vi "Analysis_Main.vi"() -> ()   [LabVIEW 2018]
uses:
  <vilib>/Utility/file.llb/Read Delimited Spreadsheet (string).vi
panel:
  in  "Path":path
  out "Duty":dbl format="%#_g %"
  out "Frequency":dbl format="%#_g Hz"
  out "DeltaT":dbl format="%#_g ms"
  in  "stop":bool
  out "Cursor 2":dbl
  out "Cursor 1":dbl
  out "Data":waveform(dbl)[](graph)
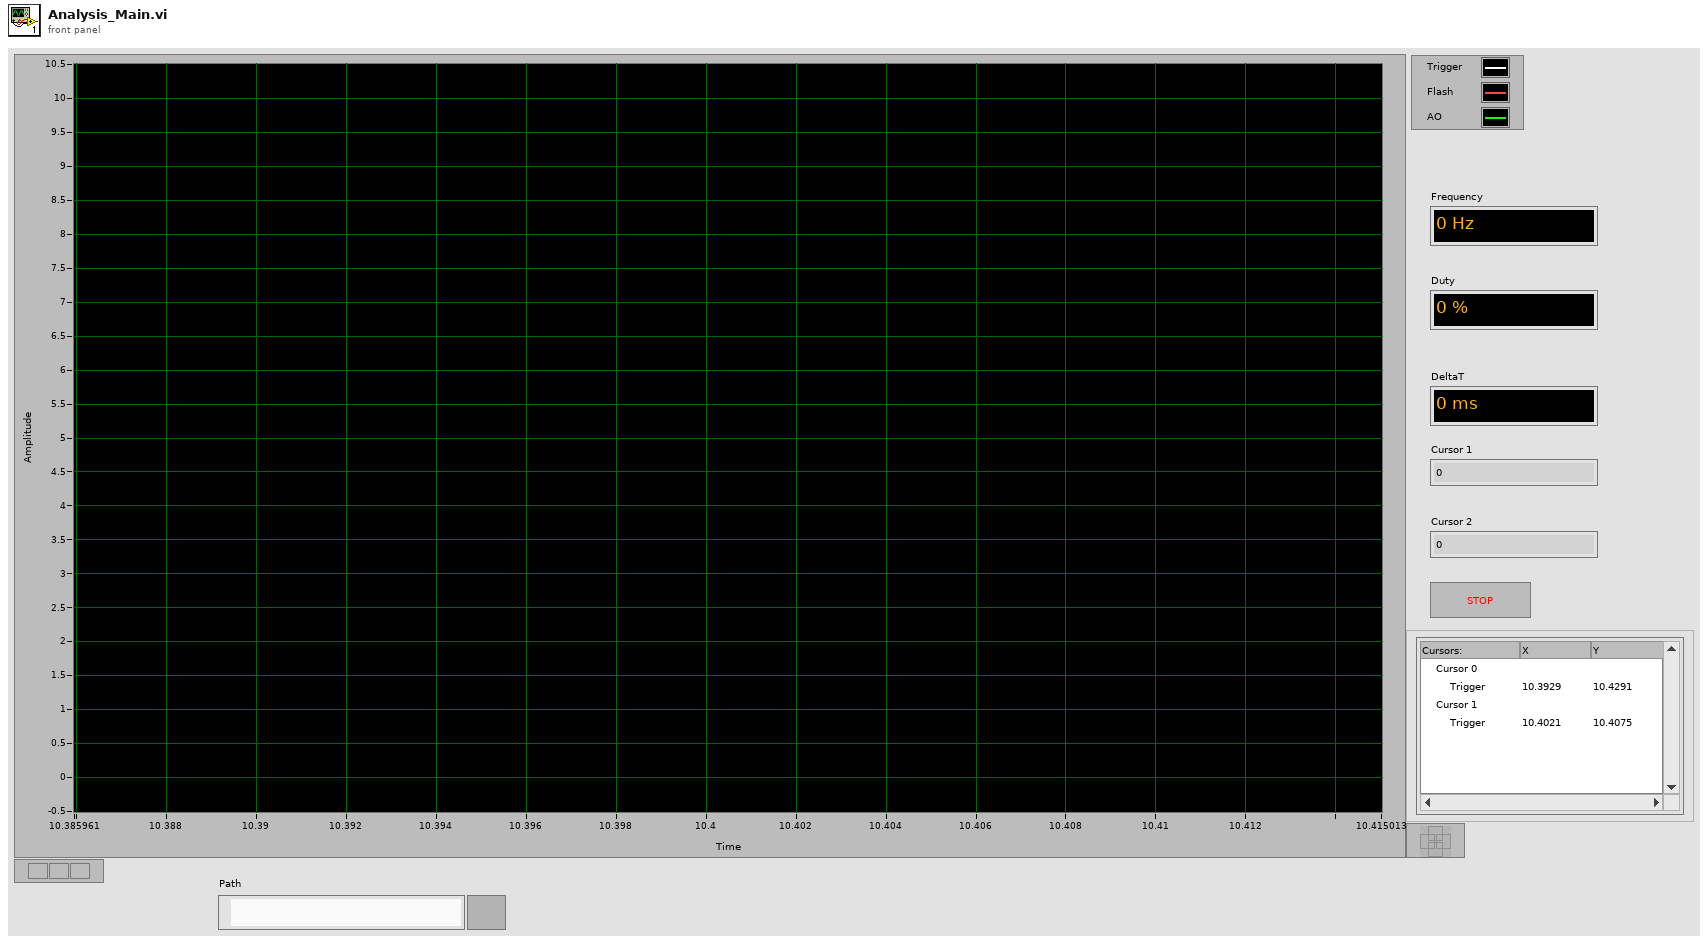
[diagram p1: front panel]
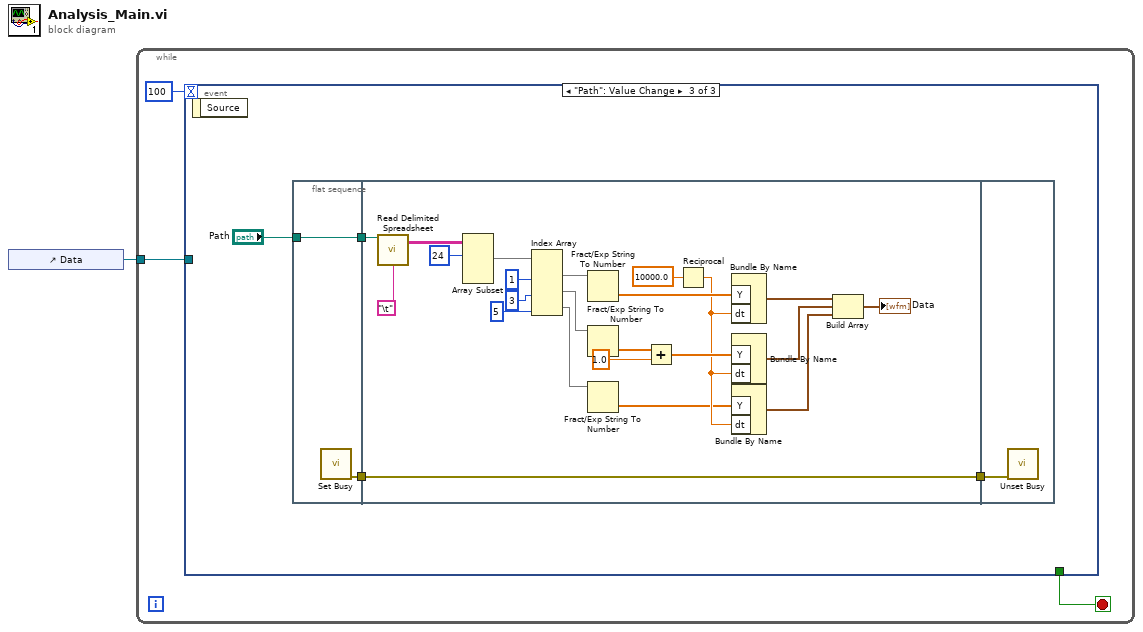
[diagram p0: block diagram]
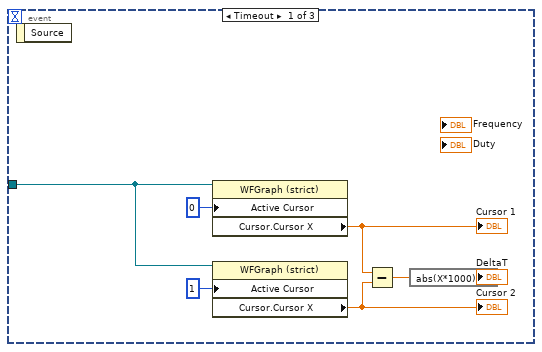
[diagram p2: hidden frame]
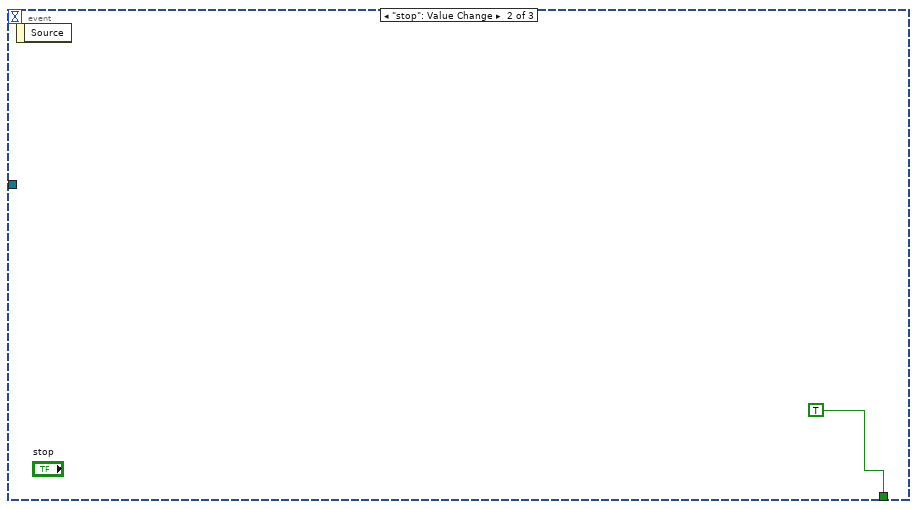
[diagram p3: hidden frame]
diagram:
  n1 = control-ref of="Data"() -> (w1:refnum<vi>)
  n2 = while {
    tunnel: w1 -> [w2]
    stop <- w4 stop-if-true
    n3 = event shown="[2] \"Path\": Value Change" {
      selector: _ -> [_ _ _]
      dyn-events: _ -> [_ _ _]
      timeout: 100 -> [_ _ _]
      tunnel: [_ TRUE _] -> w4
      tunnel: w2 -> [w5 _ _]
      event Timeout {
        n4 = event-data() -> ()  [unwired: 1 in, 1 out]
        n5 = property class="WFGraph (strict)"(reference=w5, "Active Cursor"=u32 0) -> ("Cursor.Cursor X"=w11:dbl)  [unwired: 1 in, 2 out]
        "Cursor 1" <- w11
        n6 = property class="WFGraph (strict)"(reference=w5, "Active Cursor"=u32 1) -> ("Cursor.Cursor X"=w10:dbl)  [unwired: 1 in, 2 out]
        "Cursor 2" <- w10
        n7 = Subtract(x=w11, y=w10) -> (x-y=w9:dbl)
        n8 = expression code="abs(X*1000)"(w9) -> (→"DeltaT":dbl)
      }
      event "stop": Value Change {
        n9 = event-data() -> ()  [unwired: 1 in, 1 out]
      }
      event "Path": Value Change {
        n10 = event-data() -> ()  [unwired: 1 in, 1 out]
        n11 = flat-sequence {
          tunnel: "Path" -> [w18]
          tunnel: [w18] -> w15
          tunnel: [w17] -> w14
          tunnel: w15 -> [w41]
          tunnel: w14 -> [w24]
          tunnel: [w24] -> w13
          tunnel: w13 -> [w42]
          frame #0 {
            n12 = call <vilib>:"Set Busy.vi"() -> ("error out"=w17:errorcluster)  [unwired: 10 in, 1 out]
          }
          frame #1 {
            n13 = call-poly <vilib>:"Read Delimited Spreadsheet.vi"("file path (dialog if empty)"=w41, "delimiter (\\t)"="\t") -> ("all rows"=w40:string[][])  [unwired: 8 in, 5 out]
            n14 = Array Subset(array=w40, index (row)=24 ("index")) -> (w31:string[][])  [unwired: 3 in]
            n15 = Index Array(array=w31, index (col) #1=1 ("disabled index (col)"), index (col) #2=3 ("index (col)"), index (col) #3=5 ("index (col)")) -> (element #1=w32:string[], element #2=w33:string[], element #3=w22:string[])  [unwired: 3 in]
            n16 = Fract/Exp String To Number(string=w32) -> (number=w39:dbl[])  [unwired: 3 in, 1 out]
            n17 = Fract/Exp String To Number(string=w33) -> (number=w34:dbl[])  [unwired: 3 in, 1 out]
            n18 = Fract/Exp String To Number(string=w22) -> (number=w19:dbl[])  [unwired: 3 in, 1 out]
            n19 = Add(x=w34, y=1.0) -> (x+y=w35:dbl[])
            n20 = Reciprocal(x=10000.0) -> (1/x=w21:dbl)
            n21 = Bundle By Name("Y"=w39, "dt"=w21) -> (w38:waveform(dbl))  [unwired: 1 in]
            n22 = Bundle By Name("Y"=w35, "dt"=w21) -> (w36:waveform(dbl))  [unwired: 1 in]
            n23 = Bundle By Name("Y"=w19, "dt"=w21) -> (w20:waveform(dbl))  [unwired: 1 in]
            n24 = Build Array(w38, w36, w20) -> (→"Data":waveform(dbl)[])
          }
          frame #2 {
            n25 = call <vilib>:"Unset Busy.vi"("error in (no error)"=w42) -> ()  [unwired: 10 in, 1 out]
          }
        }
      }
    }
  }
